vi "Spartan HTTP Get Session Status.vi"(8 "error in (no error)":errorcluster, 11 "http session":T1 {"object data"."time" format="%0.2f"}) -> (0 "error out":errorcluster, 2 "Connection Good":bool, 3 "http session out":T1 {"object data"."time" format="%0.2f"})   [LabVIEW 2011]
uses:
  Spartan HTTP Session.ctl
  Addons/internet/http/http_obj.llb/HTTP Session Data.ctl
  Addons/internet/utils/keyedarr.llb/Keyed Array.ctl
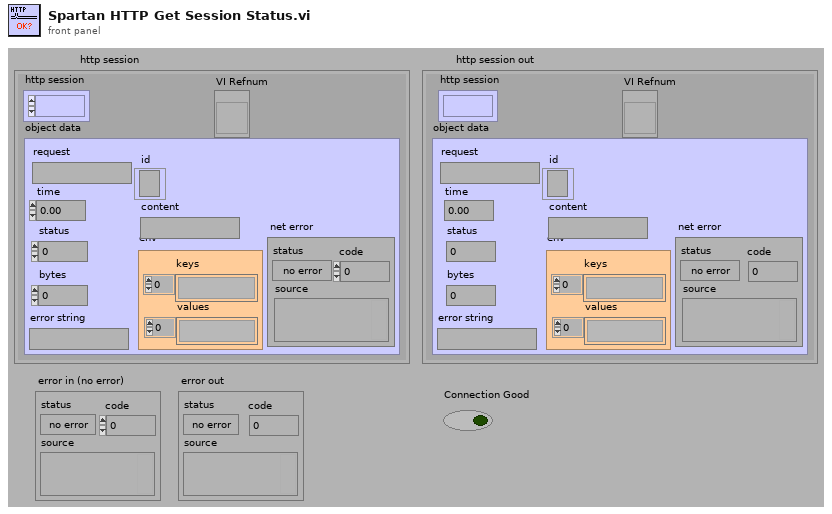
[diagram p1: front panel]
types:
  T1 = typedef "Spartan HTTP Session.ctl" = cluster{"http session":refnum<k1>, "object data":T2, "VI Refnum":refnum<vi>}
  T2 = typedef "HTTP Session Data.ctl" = cluster{"request":string, "time":dbl, "status":i32, "error string":string, "bytes":i32, "env":T3, "content":string, "id":refnum<k5>, "net error":errorcluster}
  T3 = typedef "Keyed Array.ctl" = cluster{"keys":string[], "values":string[]}
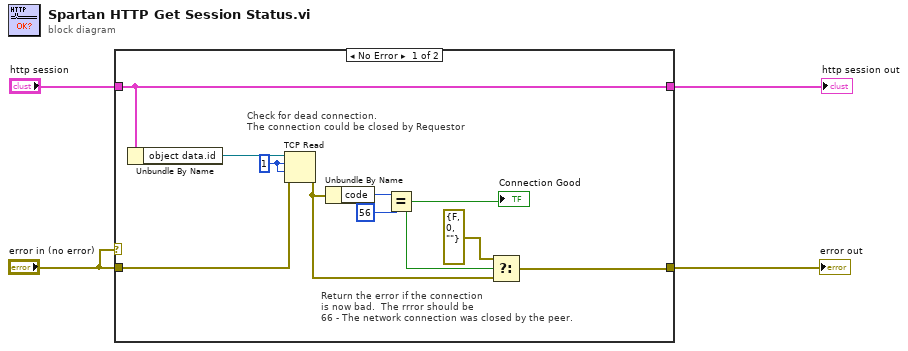
[diagram p0: block diagram]
diagram:
  n1 = case shown="No Error" "error in (no error)" {
    tunnel: "http session" -> [w5 w15]
    tunnel: [w8 w16] -> w3
    tunnel: "error in (no error)" -> [w7 w16]
    tunnel: [w5 w15] -> w1
    frame No Error {
      w13 = 1 ("bytes to read")
      # "Return the error if the connection \nis now bad.  The rrror should be\n66 - The network connection was closed by the peer."
      # "Check for dead connection.\nThe connection could be closed by Requestor"
      n2 = Unbundle By Name(w5) -> ("object data.id"=w14:refnum<k5>)
      n3 = TCP Read(connection ID=w14, bytes to read=w13, error in (no error)=w7, 9:w13) -> (error out=w9:errorcluster)  [unwired: 3 out]
      n4 = Unbundle By Name(w9) -> ("code"=w12:i32)
      n5 = Equal?(x=w12, y=56) -> (x = y?=w10:bool)
      "Connection Good" <- w10
      n6 = Select(t=errorcluster {"status"=FALSE, "code"=0, "source"=""}, s=w10, f=w9) -> (s? t:f=w8:errorcluster)
    }
    frame Error {
      # "Bypass Check on Error in"
    }
  }
  "error out" <- w3
  "http session out" <- w1
